vi "UpdateChannelsList.vi"(8 "error in (no error)":errorcluster, 10 "Channels":T1, 11 "ByteQXAPIBase in":refnum<class "ByteQXAPIBase.lvclass">) -> (0 "error out":errorcluster, 3 "ByteQXAPIBase out":refnum<class "ByteQXAPIBase.lvclass">)   [LabVIEW 2019, in "ByteQXWebAPI.lvlib" / "ByteQXAPIBase.lvclass"]
uses:
  ByteQXAPIBase.lvclass
  ChannelsList_Data.ctl
  Private/module.ctl
  ByteQXAPIBase.lvclass/ByteQXAPIBase.ctl
  <vilib>/Bytelabs/ByteREST/ByteRESTClass/ByteRESTBase/RESTBase.lvclass
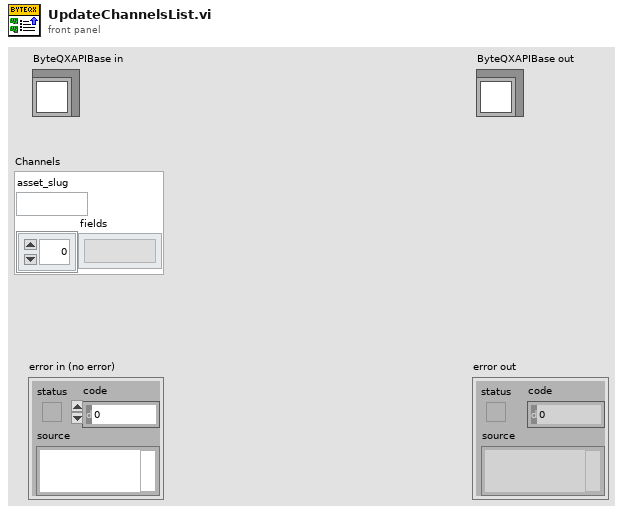
[diagram p1: front panel]
types:
  T1 = typedef "ByteQXWebAPI.lvlib/ByteQXAPIBase.lvclass/ChannelsList_Data.ctl" = cluster{"asset_slug":string, "fields":string[]}
  T2 = typedef "ByteQXWebAPI.lvlib/ByteQXAPIBase.lvclass/module.ctl" = enum16{"gs", "tms"}
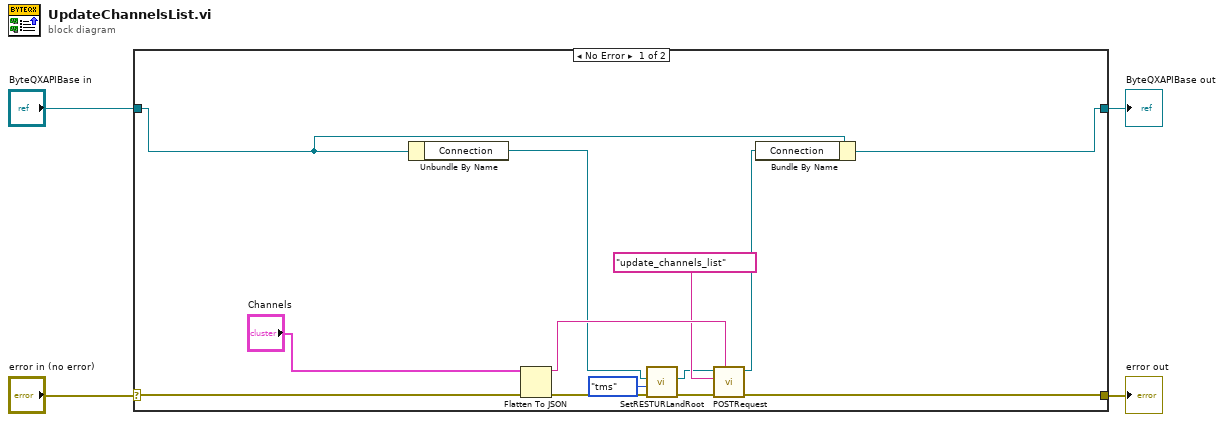
[diagram p0: block diagram]
diagram:
  n1 = case shown="No Error" "error in (no error)" {
    selector: "error in (no error)" -> [w14 w19]
    tunnel: [w13 w19] -> w3
    tunnel: [w10 w18] -> w1
    tunnel: "ByteQXAPIBase in" -> [w11 w18]
    frame No Error {
      n2 = Unbundle By Name(w11) -> ("Connection"=w7:refnum<class "RESTBase.lvclass">)
      n3 = Flatten To JSON(anything="Channels", error in (no error)=w14) -> (JSON string=w17:string, 11:w9:errorcluster)  [unwired: 1 in]
      n4 = call "SetRESTURLandRoot.vi"("error in (no error)"=w9, "module"=module."tms", "ByteREST in"=w7) -> ("error out"=w8:errorcluster, "ByteREST out"=w6:refnum<class "RESTBase.lvclass">)  [unwired: 7 in]
      n5 = call-dynamic "POSTRequest.vi"("Body in"=w17, "error in (no error)"=w8, "Request"="update_channels_list", "ByteRESTBase in"=w6) -> ("error out"=w13:errorcluster, "ByteRESTBase out"=w16:refnum<class "RESTBase.lvclass">)  [unwired: 4 in, 2 out]
      n6 = Bundle By Name(cluster=w11, "Connection"=w16) -> (w10:refnum<class "ByteQXAPIBase.lvclass">)
    }
    frame Error {
    }
  }
  "error out" <- w3
  "ByteQXAPIBase out" <- w1
